vi "Pod Code.vi"() -> ()   [LabVIEW 2014]
uses:
  Type Defs/Relays.ctl
  Type Defs/SensorStates.ctl
  Sensors/Time of Flight - VL6180/VL6180 Resource.ctl
  <vilib>/Platform/TimedLoop/XDataNode/timing_clust.ctl
  <vilib>/Platform/TimedLoop/XDataNode/nitl_modes.ctl
  <vilib>/Platform/TimedLoop/XDataNode/wakeup.ctl
  <vilib>/myRIO/Instrument Drivers/Onboard Devices/Accelerometer/typedefs/Accelerometer Reference.ctl
  <vilib>/myRIO/Common/Instrument Driver Framework/Utilities/typedefs/myRIO Generic Hardware Reference.ctl
  <vilib>/myRIO/Common/Instrument Driver Framework/Utilities/typedefs/Hardware Version Enum.ctl
  <vilib>/myRIO/Common/Instrument Driver Framework/Utilities/typedefs/myRIO v1.0 Reference.ctl
  <vilib>/myRIO/Common/Instrument Driver Framework/Utilities/typedefs/Generic FPGA Reference.ctl
  <vilib>/myRIO/Common/Instrument Driver Framework/myRIO v1.0/Accelerometer/typedefs/Accelerometer Channels List.ctl
  <vilib>/myRIO/Common/Instrument Driver Framework/myRIO v1.0/Accelerometer/typedefs/Accelerometer Channels Enum.ctl
  <vilib>/userdefined/High Color/nirio_resource_hc.ctl
  <vilib>/myRIO/Instrument Drivers/Onboard IO/DIO/typedefs/DIO Reference.ctl
  <vilib>/myRIO/Common/Instrument Driver Framework/myRIO v1.0/DIO/typedefs/DIO Channels List.ctl
  <vilib>/myRIO/Common/Instrument Driver Framework/myRIO v1.0/DIO/typedefs/DIO Channels Enum.ctl
  <vilib>/myRIO/Common/Instrument Driver Framework/Utilities/vis/Is FPGA Ref Available.vi
  <vilib>/myRIO/Common/Instrument Driver Framework/myRIO v1.0/Accelerometer/vis/myRIO v1.1 Open Accelerometer.vi
  <vilib>/myRIO/Instrument Drivers/Onboard Devices/Accelerometer/vis/Read.vi
  <vilib>/myRIO/Common/Instrument Driver Framework/myRIO v1.0/DIO/vis/myRIO v1.1 Open DIO.vi
  <vilib>/myRIO/Instrument Drivers/Onboard IO/DIO/vis/Read.vi
  <vilib>/myRIO/Instrument Drivers/Onboard IO/DIO/vis/Write.vi
  <vilib>/myRIO/Common/Instrument Driver Framework/Utilities/vis/Validate Channels.vi
  <vilib>/myRIO/Common/Instrument Driver Framework/myRIO v1.0/Accelerometer/vis/myRIO v1.0 Reserve Accelerometer.vi
  <vilib>/myRIO/Common/Instrument Driver Framework/myRIO v1.0/DIO/vis/myRIO v1.0 Reserve DIO.vi
  <vilib>/myRIO/Common/Instrument Driver Framework/myRIO v1.0/Resource Manager/vis/myRIO v1.0 Reserve Channel List.vi
  <vilib>/myRIO/Common/Instrument Driver Framework/myRIO v1.0/Accelerometer/vis/myRIO v1.0 Build MUX Configuration Accelerometer.vi
  <vilib>/myRIO/Common/Instrument Driver Framework/myRIO v1.0/DIO/vis/myRIO v1.0 Build MUX Configuration DIO.vi
  <vilib>/myRIO/Common/Instrument Driver Framework/myRIO v1.0/Resource Manager/vis/myRIO v1.0 Reserve Channel.vi
  <vilib>/myRIO/Common/Instrument Driver Framework/myRIO v1.0/Resource Manager/vis/myRIO v1.0 Unreserve Channel.vi
  <vilib>/myRIO/Common/Instrument Driver Framework/myRIO v1.0/Resource Manager/vis/myRIO v1.0 Create Configuration List.vi
  <vilib>/myRIO/Common/Instrument Driver Framework/myRIO v1.0/Resource Manager/vis/myRIO v1.0 Build Mutex Name.vi
  <vilib>/Utility/VariantDataType/GetNumericInfo.vi
  <vilib>/Utility/error.llb/Error Cluster From Error Code.vi
  <vilib>/myRIO/Common/Instrument Driver Framework/myRIO v1.0/myRIO v1.1 Open.vi
  <vilib>/myRIO/Common/Instrument Driver Framework/Utilities/vis/IO Manager.vi
  <vilib>/myRIO/Common/Instrument Driver Framework/Utilities/vis/Configuration Manager.vi
  <vilib>/myRIO/Common/Instrument Driver Framework/myRIO v1.0/Resource Manager/vis/myRIO v1.0 Configure IO.vi
  <vilib>/myRIO/Common/Instrument Driver Framework/myRIO v1.0/myRIO v1.0 Close.vi
  <vilib>/myRIO/Common/Instrument Driver Framework/myRIO v1.0/DIO/vis/myRIO v1.0 Write DIO.vi
  <vilib>/myRIO/Common/Instrument Driver Framework/myRIO v1.0/Accelerometer/vis/myRIO v1.0 Get Scaling Constant Accelerometer.vi
  <vilib>/myRIO/Common/Instrument Driver Framework/myRIO v1.0/Accelerometer/vis/myRIO v1.0 Read Accelerometer.vi
  <vilib>/myRIO/Common/Instrument Driver Framework/myRIO v1.0/DIO/vis/myRIO v1.0 Read DIO.vi
  <vilib>/myRIO/Express VI/Onboard IO/DO/DO Express VI.xnode
  <vilib>/myRIO/Instrument Drivers/Onboard IO/DIO/vis/myRIO DIO Open.xnode
  <vilib>/platform/TimedLoop/XDataNode/XDataNode.xnode
  <vilib>/myRIO/Express VI/Onboard Devices/Accelerometer/Accelerometer Express VI.xnode
  <vilib>/myRIO/Instrument Drivers/Onboard Devices/Accelerometer/vis/myRIO Accelerometer Open.xnode
  <vilib>/myRIO/Express VI/Onboard IO/DI/DI Express VI.xnode
  <vilib>/myRIO/Instrument Drivers/Onboard IO/DIO/DIO.lvlib
  <vilib>/MakerHub/LINX/LMH-LINX.lvlib
  <vilib>/Platform/TimedLoop/XDataNode/XDNodeRunTimeDep.lvlib
  <vilib>/myRIO/Instrument Drivers/Onboard Devices/Accelerometer/Accelerometer.lvlib
panel:
  out "Laser Error":bool
  out "Accelerometer Error":bool
  in  "Reset Count":bool
  out "Laser 1 Count":u32
  out "Laser 2 Count":u32
  out "Fancy Laser Count":u32
  out "Back":dbl
  out "Right":dbl
  out "Up":dbl
  out "Laser 1":bool
  out "Laser 2":bool
  out "Laser 3":bool
  in  "Fire Z Lasers!":bool
  out "Pressure Readings (PSI)":dbl[](array[numeric])
  in  "ToFs":T1[](array[typedef])=[enum."ToF1", enum."ToF2", enum."ToF3", enum."ToF5"]
  out "Sensor Error":errorcluster
  out "ToF Online":bool[](array[boolean])
  in  "Reset Sensors":bool
  out "Distance Readings":u8[](array[numeric])
  out "Actuator Error":errorcluster
  in  "Stop Button":bool
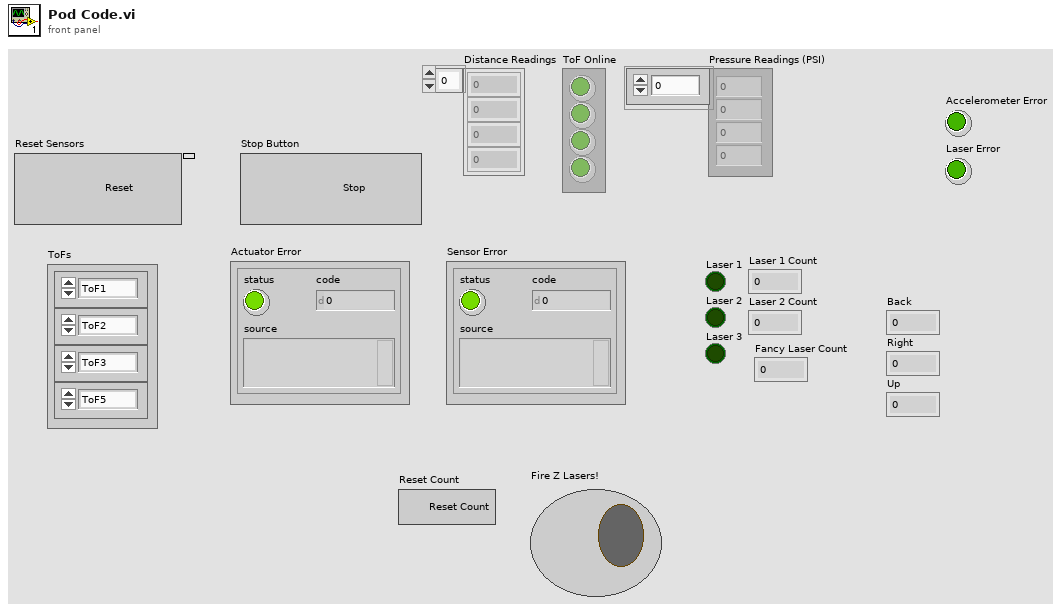
[diagram p1: front panel]
types:
  T1 = typedef "Relays.ctl" = enum16{"ToF1", "ToF2", "ToF3", "ToF4", "ToF5", "ToF6", "ToF7", "ToF8", "SensePwr", "All"}
  T2 = typedef "VL6180 Resource.ctl" = cluster{"I2C Channel":u8, "I2C Slave Address":u8, "Online":bool}
  T3 = typedef "SensorStates.ctl" = enum16{"Reset", "Read", "Close"}
  T4 = typedef "LMH-LINX.lvlib/LINX Ref.ctl" = cluster{"IO":T5, "Interface":T6, "LINX Device Config":T7}
  T5 = typedef "LMH-LINX.lvlib/Platform.ctl" = enum16{"Remote", "Local"}
  T6 = typedef "LMH-LINX.lvlib/Interface.ctl" = enum16{"Serial", "TCP"}
  T7 = typedef "LMH-LINX.lvlib/Device.lvlib/LINX Device Config.ctl" = cluster{"Interface":T6, "COM Port":refnum<visa-resource-name>, "TCP Configuration":T8, "Device Family":u8, "Device ID":u8, "Device Name":string, "TCP Ref":refnum<k5>, "Channels":T9}
  T8 = typedef "LMH-LINX.lvlib/Device.lvlib/TCP Config.ctl" = cluster{"IP Address":string, "Port":u16}
  T9 = typedef "LMH-LINX.lvlib/Channels.ctl" = cluster{"DI":u8[], "DO":u8[], "AI":u8[], "AO":u8[], "PWM":u8[], "QE":u8[], "UART":u8[], "I2C 2":u8[], "SPI":u8[], "CAN":u8[], "Servo":u8[], "AI Ref (V)":dbl, "AI Resolution (Bits)":u8, "AO Ref (V)":dbl, "AO Resolution (Bits)":u8}
  T10 = typedef "XDNodeRunTimeDep.lvlib/timing_clust.ctl" = cluster{"Expected End [f-1]":u64, "Actual End [f-1]":u64, "Finished Late? [f-1]":bool, "Expected End [i-1]":u64, "Actual End [i-1]":u64, "Finished Late? [i-1]":bool, "Expected Start [i]":u64, "Actual Start [i]":u64, "Expected Start [f]":u64, "Actual Start [f]":u64, "Source Name":string, "Structure Name":string, "Period":i64, "Deadline":i64, "Offset":i64, "Start":i64, "Priority":i32, "Timeout":i32, "Mode":T11, "Wakeup Reason":T12, "Error":errorcluster, "Source Type":string, "Secondary Source Type":string, "Global End Time":u64, "Global Start Time":u64, "Frame Duration":u64, "Iteration Duration":u64, "Assigned CPU":i32, "I/O Scan Engine Mode":u32}
  T11 = typedef "XDNodeRunTimeDep.lvlib/nitl_modes.ctl" = enum32{"No Change", "Process missed periods, maintain original phase", "Discard missed periods, maintain original phase", "Process missed periods, ignore original phase", "Discard missed periods, ignore original phase"}
  T12 = typedef "XDNodeRunTimeDep.lvlib/wakeup.ctl" = enum32{"Normal", "Aborted", "Asynchronous wakeup", "Timing source error", "Timed loop error", "Timeout"}
  T13 = typedef "DIO.lvlib/DIO Reference.ctl" = cluster{"myRIO Reference":T14, "DIO Channels List":T18}
  T14 = typedef "myRIO Generic Hardware Reference.ctl" = cluster{"myRIO Model":T15, "myRIO Hardware Reference":T16}
  T15 = typedef "Hardware Version Enum.ctl" = enum16{"Unknown", "myRIO-1900", "myRIO-1950"}
  T16 = typedef "myRIO v1.0 Reference.ctl" = cluster{"Generic FPGA Reference":T17, "Allow multiple opens":bool}
  T17 = typedef "Generic FPGA Reference.ctl" = refnum<k20>
  T18 = typedef "DIO Channels List.ctl" = T19[]
  T19 = typedef "DIO Channels Enum.ctl" = enum16{"Not Connected", "C/DIO0", "C/DIO1", "C/DIO2", "C/DIO3", "C/DIO4", "C/DIO5", "C/DIO6", "C/DIO7", "A/DIO0", "A/DIO1", "A/DIO2", "A/DIO3", "A/DIO4", "A/DIO5", "A/DIO6", "A/DIO7", "A/DIO8", "A/DIO9", "A/DIO10", "A/DIO11", "A/DIO12", "A/DIO13", "A/DIO14", "A/DIO15", "B/DIO0", "B/DIO1", "B/DIO2", "B/DIO3", "B/DIO4", "B/DIO5", "B/DIO6", "B/DIO7", "B/DIO8", "B/DIO9", "B/DIO10", "B/DIO11", "B/DIO12", "B/DIO13", "B/DIO14", "B/DIO15", "LED0", "LED1", "LED2", "LED3", "Button0"}
  T20 = typedef "nirio_resource_hc.ctl" = tag
  T21 = typedef "Accelerometer.lvlib/Accelerometer Reference.ctl" = cluster{"myRIO Reference":T14, "Accelerometer Channels List":T22, "LSB Weight":dbl}
  T22 = typedef "Accelerometer Channels List.ctl" = T23[]
  T23 = typedef "Accelerometer Channels Enum.ctl" = enum16{"Not Connected", "X-Axis", "Y-Axis", "Z-Axis"}
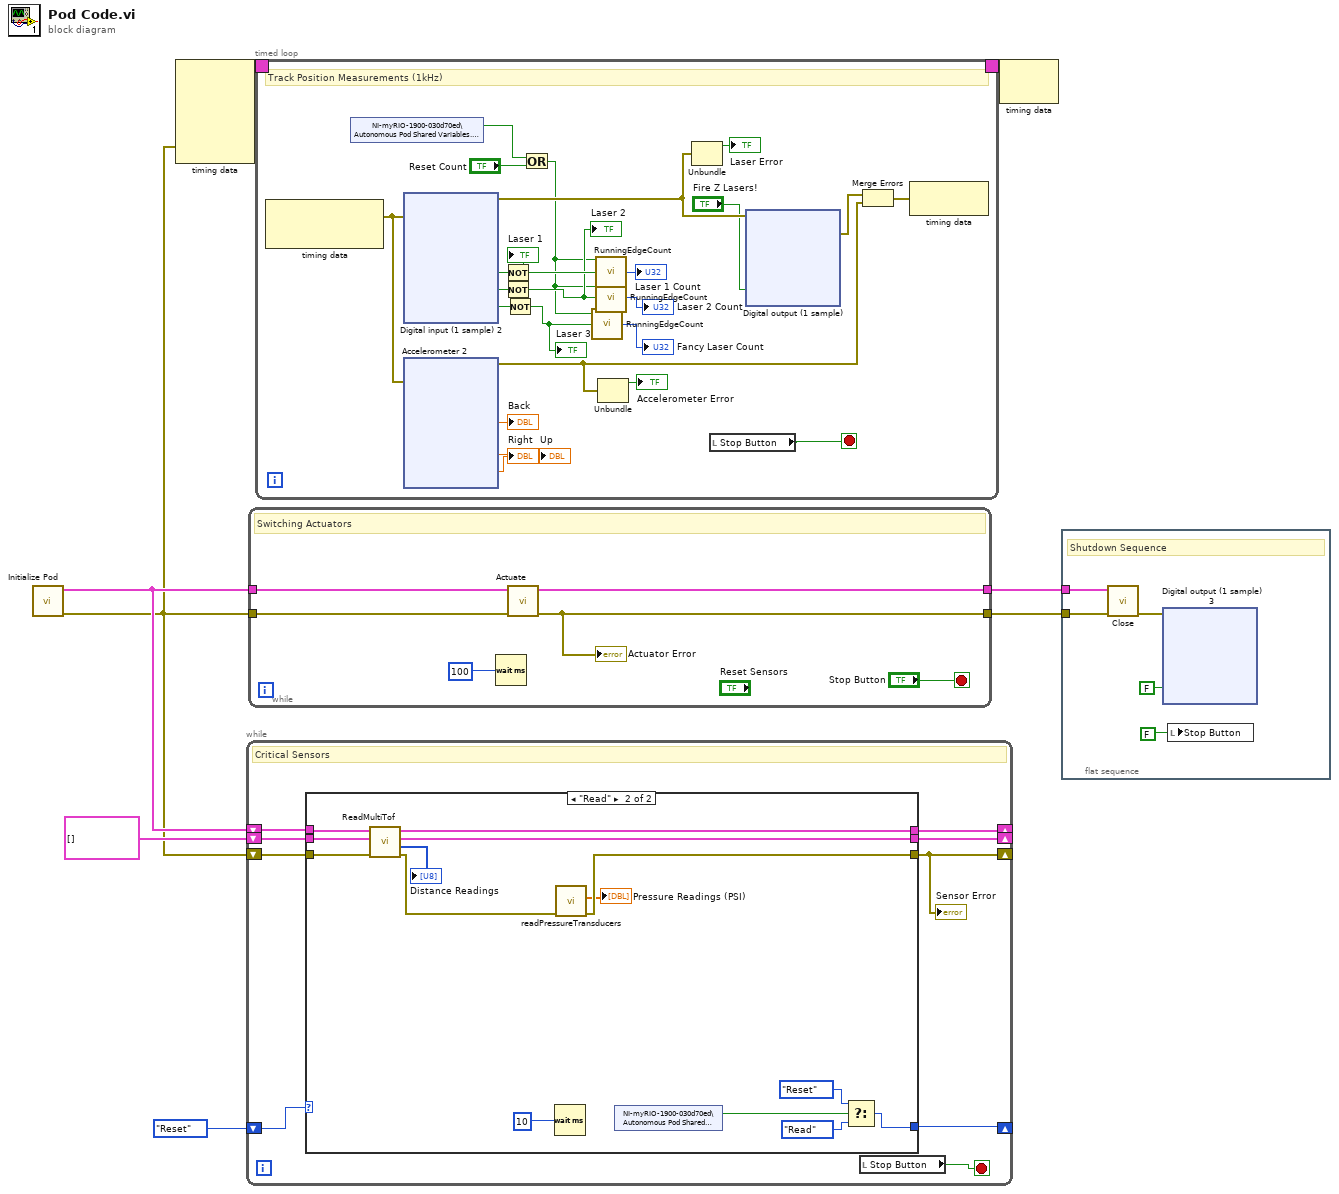
[diagram p0: block diagram]
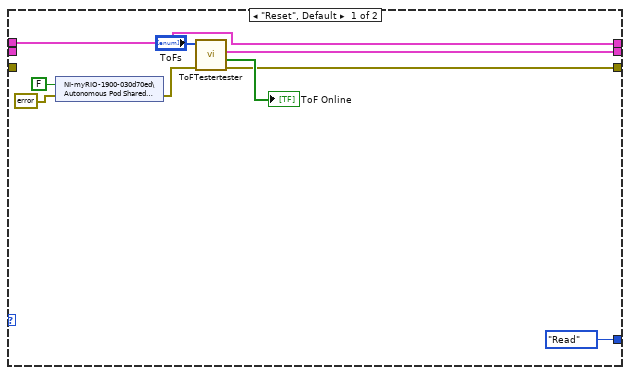
[diagram p2: hidden frame]
diagram:
  n1 = call "Initialize Pod.vi"() -> ("error out"=w1:errorcluster, "LINX Resource"=w5:T4)  [unwired: 10 in]
  n2 = node-c288(w1) -> (w3:T10)  [unwired: 4 in]
  n3 = while {
    shift-right: [w15] -> _
    shift-left: SensorStates."Reset" -> [w17]
    shift-right: [w9] -> _
    shift-left: w1 -> [w16]
    shift-right: [w12] -> _
    shift-left: w5 -> [w14]
    shift-right: [w11] -> _
    shift-left: T2[] [] ("VL Configs") -> [w10]
    stop <- w13 stop-if-true
    # "Critical Sensors"
    n4 = case shown="\"Read\"" w17 {
      tunnel: w16 -> [_ w34]
      tunnel: [w22 w28] -> w9
      tunnel: [SensorStates."Read" w39] -> w15
      tunnel: w14 -> [w24 w35]
      tunnel: [w24 w33] -> w12
      tunnel: [w25 w32] -> w11
      tunnel: w10 -> [_ w36]
      frame "Reset", Default {
        n5 = shared-variable "NI-myRIO-1900-030d70ed\\Autonomous Pod Shared Variables.lvlib\\ResetSensor"(FALSE ("ResetSensor"), error in=errorcluster {"status"=FALSE, "code"=0, "source"=""}) -> (error out=w20:errorcluster)
        n6 = call "ToFTestertester.vi"("error in"=w20, "ToFs"="ToFs") -> ("error out"=w22:errorcluster, "ToF Online"=→"ToF Online":bool[], "ToF Details"=w25:T2[])  [unwired: 7 in]
      }
      frame "Read" {
        n7 = call "ReadMultiTof.vi"("error in"=w34, "VL6180 Resources"=w36, "LINX Resource in"=w35) -> ("error out"=w29:errorcluster, "Distance Readings"=→"Distance Readings":u8[], "VL Configs"=w32:T2[], "LINX Resource out"=w33:T4)  [unwired: 5 in]
        n8 = Wait (ms)(milliseconds to wait=u32 10) -> ()  [unwired: 1 out]
        n9 = call "readPressureTransducers.vi"("error in"=w29) -> ("error out"=w28:errorcluster, "Pressure Readings"=→"Pressure Readings (PSI)":dbl[])  [unwired: 9 in]
        n10 = shared-variable "NI-myRIO-1900-030d70ed\\Autonomous Pod Shared Variables.lvlib\\ResetSensor"() -> (w30:bool)  [unwired: 1 in, 1 out]
        n11 = Select(t=SensorStates."Reset", s=w30, f=SensorStates."Read") -> (s? t:f=w39:T3)
      }
    }
    "Sensor Error" <- w9
    n12 = local read "Stop Button"() -> (w13:bool)
  }
  n13 = while {
    tunnel: w5 -> [w44]
    tunnel: [w43] -> w8
    tunnel: [w41] -> w7
    tunnel: w1 -> [w42]
    stop <- "Stop Button" stop-if-true
    # "Switching Actuators"
    n14 = Wait (ms)(milliseconds to wait=u32 100) -> ()  [unwired: 1 out]
    n15 = call "Actuate.vi"("error in (no error)"=w42, "LINX Resource in"=w44) -> ("error out"=w41:errorcluster, "LINX Resource out"=w43:T4)  [unwired: 7 in, 1 out]
    "Actuator Error" <- w41
  }
  n16 = timed-loop {
    timing: w3 -> [_]
    timing-out: [_] -> w2
    stop <- w47 stop-if-true
    # "Track Position Measurements (1kHz)"
    n17 = node-c288() -> (w66:errorcluster)  [unwired: 1 in, 1 out]
    n18 = shared-variable "NI-myRIO-1900-030d70ed\\Autonomous Pod Shared Variables.lvlib\\ResetLaserCount"() -> (w50:bool)  [unwired: 1 in, 1 out]
    n19 = xnode "Digital input (1 sample) 2"("error in (no error)"=w66) -> ("Laser 1 (B/DIO9 (Pin 29))"=w64:bool, "Laser 2 (B/DIO10 (Pin 31))"=w65:bool, "Fancy Laser (B/DIO11 (Pin 18))"=w62:bool, "error out"=w53:errorcluster)
    n20 = xnode "Accelerometer 2"("error in (no error)"=w66) -> ("Back"=→"Back":dbl, "Right"=→"Right":dbl, "Up"=→"Up":dbl, "error out"=w70:errorcluster)
    n21 = Not(x=w64) -> (.not. x?=w68:bool)
    "Laser 1" <- w68
    n22 = Not(x=w65) -> (.not. x?=w55:bool)
    "Laser 2" <- w55
    n23 = Not(x=w62) -> (.not. x?=w54:bool)
    "Laser 3" <- w54
    n24 = Or(x=w50, y="Reset Count") -> (x .or. y?=w48:bool)
    n25 = call "RunningEdgeCount.vi"("Reset Count? (F)"=w48, "Input"=w54) -> ("Count"=→"Fancy Laser Count":u32)  [unwired: 3 in]
    n26 = call "RunningEdgeCount.vi"("Reset Count? (F)"=w48, "Input"=w68) -> ("Count"=→"Laser 1 Count":u32)  [unwired: 3 in]
    n27 = call "RunningEdgeCount.vi"("Reset Count? (F)"=w48, "Input"=w55) -> ("Count"=→"Laser 2 Count":u32)  [unwired: 3 in]
    n28 = Unbundle(w70) -> ("status"=→"Accelerometer Error":bool)  [unwired: 2 out]
    n29 = Unbundle(w53) -> ("status"=→"Laser Error":bool)  [unwired: 2 out]
    n30 = local read "Stop Button"() -> (w47:bool)
    n31 = xnode "Digital output (1 sample)"("Sense Power (B/DIO8 (Pin 27))"="Fire Z Lasers!", "error in (no error)"=w53) -> ("error out"=w52:errorcluster)
    n32 = Merge Errors(w52, w70) -> (w63:errorcluster)
    n33 = node-c288(w63) -> ()  [unwired: 1 out]
  }
  n34 = node-c288(w2) -> ()  [unwired: 1 out]
  n35 = flat-sequence {
    tunnel: w8 -> [w190]
    tunnel: w7 -> [w189]
    frame #0 {
      # "Shutdown Sequence"
      n36 = call <vilib>:"Close.vi"("Error In"=w189, "LINX Resource"=w190) -> ("Error Out"=w188:errorcluster)  [unwired: 9 in]
      n37 = xnode "Digital output (1 sample) 3"("Activate Pneumatics (A/DIO10 (Pin 31))"=FALSE ("Levitation"), "error in (no error)"=w188) -> ()  [unwired: 1 out]
      n38 = local write "Stop Button"(FALSE ("Stop Button")) -> ()
    }
  }
